vi "Write Model.vi"(8 "error in (no error)":errorcluster, 10 "Model":string, 11 "GEN40-38-LAN in":refnum<class "GEN40-38-LAN.lvclass">) -> (0 "error out":errorcluster, 3 "GEN40-38-LAN out":refnum<class "GEN40-38-LAN.lvclass">)   [LabVIEW 2018, in "GEN40-38-LAN.lvlib" / "GEN40-38-LAN.lvclass"]
uses:
  GEN40-38-LAN.lvclass
  GEN40-38-LAN.lvclass/GEN40-38-LAN.ctl
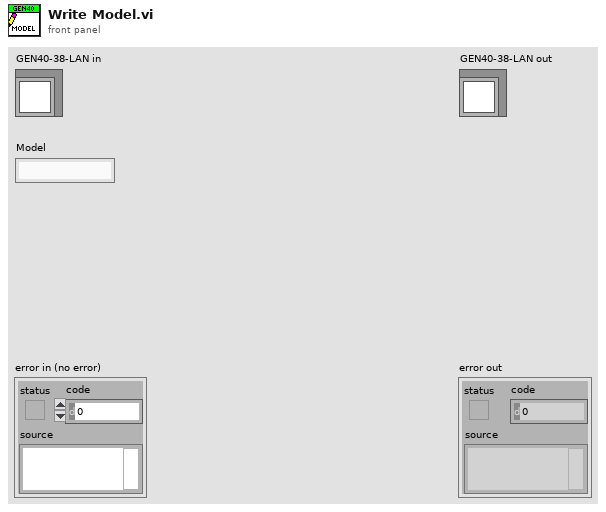
[diagram p1: front panel]
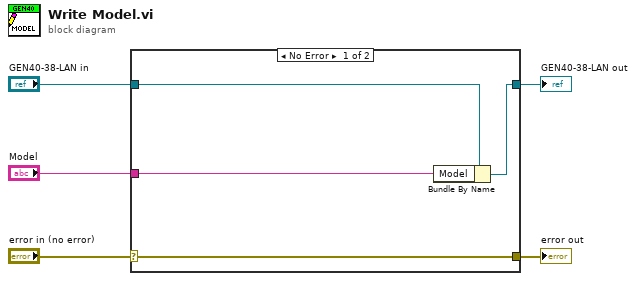
[diagram p0: block diagram]
diagram:
  n1 = case shown="No Error" "error in (no error)" {
    selector: "error in (no error)" -> [w9 w10]
    tunnel: [w9 w10] -> w4
    tunnel: [w7 w11] -> w2
    tunnel: "GEN40-38-LAN in" -> [w8 w11]
    tunnel: "Model" -> [w6 _]
    frame No Error {
      n2 = Bundle By Name(cluster=w8, "Model"=w6) -> (w7:refnum<class "GEN40-38-LAN.lvclass">)
    }
    frame Error {
    }
  }
  "error out" <- w4
  "GEN40-38-LAN out" <- w2
